vi "Host Access Control (SubVI).vi"(8 "Master /slave":bool, 10 "System Down?":bool, 11 "Data Cluster in":T1={"VI References"=[], "Addresses"=[], "Pilot"=FALSE, "DO Data"=[], "Access Restricted?"=FALSE, "Pilot Control References"=[], "CoPilot Control References"=[], "cRIO Config"=[], "datalog Q"=refnum, "PS_P"={"AI"=[], "DI"=[], "DO"=[], "Serial"=[], "CPU"={"Total Load"=[], "Interrupt Load"=[], "Total Physical"=0.0, "Free Physical"=0.0, "Primary Disk Capacity"=0.0, "Primary Disk Free"=0.0}, "Stop"=FALSE, "DO Channel"=[]}, "PS_S"={"AI"=[], "DI"=[], "DO"=[], "Serial"=[], "CPU"={"Total Load"=[], "Interrupt Load"=[], "Total Physical"=0.0, "Free Physical"=0.0, "Primary Disk Capacity"=0.0, "Primary Disk Free"=0.0}, "Stop"=FALSE, "DO Channel"=[]}, "IDE_P"={"AI"=[], "DI"=[], "DO"=[], "Serial"=[], "CPU"={"Total Load"=[], "Interrupt Load"=[], "Total Physical"=0.0, "Free Physical"=0.0, "Primary Disk Capacity"=0.0, "Primary Disk Free"=0.0}, "Stop"=FALSE, "DO Channel"=[]}, "IDE_S"={"AI"=[], "DI"=[], "DO"=[], "Serial"=[], "CPU"={"Total Load"=[], "Interrupt Load"=[], "Total Physical"=0.0, "Free Physical"=0.0, "Primary Disk Capacity"=0.0, "Primary Disk Free"=0.0}, "Stop"=FALSE, "DO Channel"=[]}, "PDE_P"={"AI"=[], "DI"=[], "DO"=[], "Serial"=[], "CPU"={"Total Load"=[], "Interrupt Load"=[], "Total Physical"=0.0, "Free Physical"=0.0, "Primary Disk Capacity"=0.0, "Primary Disk Free"=0.0}, "Stop"=FALSE, "DO Channel"=[]}, "PDE_S"={"AI"=[], "DI"=[], "DO"=[], "Serial"=[], "CPU"={"Total Load"=[], "Interrupt Load"=[], "Total Physical"=0.0, "Free Physical"=0.0, "Primary Disk Capacity"=0.0, "Primary Disk Free"=0.0}, "Stop"=FALSE, "DO Channel"=[]}, "GUI References"={"Control Names"=[], "Control References"=[]}, "GUI Data"=[], "TCP - Serial"=[], "TCP-Serial Q"=refnum, "TCP Serial Ref"=[], "Data Sets"=[], "Last Data"=[], "Alarm Data"=[], "DI Data"=[], "Ack Data"=[], "Buzzer Data"=[], "Pilot DO"=[], "Co-Pilot DO"=[], "System Down?"=FALSE, "Log Data"=[], "Update Array"=[], "MCC Data Log"=[], "MCC Data Not"=refnum, "Thruster control"=[refnum, refnum, refnum, refnum, refnum, refnum, refnum, refnum, refnum], "waga notifier out"=refnum, "Wago  log"=[], "Thruster Cont"=[0.0, 0.0, 0.0, 0.0, 0.0, 0.0, 0.0, 0.0, 0.0], "Cam Cont"=[FALSE, FALSE, FALSE, FALSE, FALSE, TRUE], "PDE_P TH Cont"={"COM 10"=0.0, "COM 11"=0.0, "COM 12"=0.0, "COM 13"=0.0}, "PDE_S TH Cont"={"COM 10"=0.0, "COM 11"=0.0, "COM 12"=0.0, "COM 13"=0.0}} {"cRIO Config"."AI"."Interface Data"."Timing"."sample mode" items=["Finite Samples"=10178, "Continuous Samples"=10123, "Hardware Timed Single Point"=12522]; "cRIO Config"."Async"."Interface Data"."Data"."Minor Frame Count" min=5 max=8 step=1}) -> ()   [LabVIEW 2021]
doc: "Control acess will be define here based on the Master or slave status & System Done Status which det from the Watch Dog UDP vi"
uses:
  Controls/Host - GUI Data Cluster.ctl
  Analog Output/Controls/AO JSON Data Cluster.ctl
  Analog Output/Controls/AO Interface Data Cluster.ctl
  Analog Output/Controls/AO Channel Configuration Cluster.ctl
  Analog Output/Controls/AO Timing Cluster.ctl
  Digital Output/Controls/DIO Configuration cluster.ctl
  Digital Output/Controls/DIO Interface Data.ctl
  Digital Output/SubVIs/Digital Dynamic Cluster.ctl
  Async JSON Cluster.ctl
  Async Interface Data Cluster.ctl
  Async Serial/Controls/Async Serial Configuration Cluster.ctl
  Async Serial/Controls/Async Frame Info Cluster.ctl
  Async Serial/Controls/Async Message Info Cluster.ctl
  Controls/Host Data Cluster.ctl
  Main Engine/Controls/Main Engine CPU Info.ctl
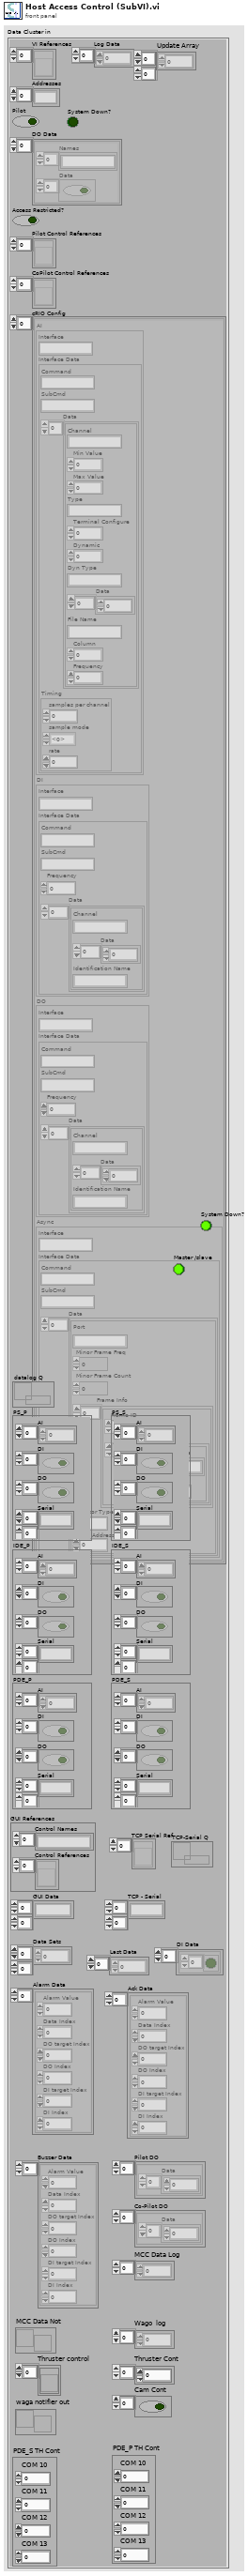
[diagram p1: front panel]
types:
  T1 = typedef "Host - GUI Data Cluster.ctl" = cluster{"VI References":refnum<vi>[], "Addresses":string[], "Pilot":bool, "DO Data":cluster{"Names":string[], "Data":bool[]}[], "Access Restricted?":bool, "Pilot Control References":refnum<vi>[], "CoPilot Control References":refnum<vi>[], "cRIO Config":cluster{"AI":T2, "DI":T6, "DO":T6, "Async":T9}[], "datalog Q":refnum<queue>, "PS_P":T14, "PS_S":T14, "IDE_P":T14, "IDE_S":T14, "PDE_P":T14, "PDE_S":T14, "GUI References":cluster{"Control Names":string[], "Control References":refnum<vi>[]}, "GUI Data":string[][], "TCP - Serial":string[][], "TCP-Serial Q":refnum<queue>, "TCP Serial Ref":refnum<vi>[], "Data Sets":dbl[][], "Last Data":dbl[], "Alarm Data":cluster{"Alarm Value":dbl, "Data Index":i32, "DO target Index":i32, "DO Index":i32, "DI target Index":i32, "DI Index":i32}[], "DI Data":cluster{bool[]}[], "Ack Data":cluster{"Alarm Value":dbl, "Data Index":i32, "DO target Index":i32, "DO Index":i32, "DI target Index":i32, "DI Index":i32}[], "Buzzer Data":cluster{"Alarm Value":dbl, "Data Index":i32, "DO target Index":i32, "DO Index":i32, "DI target Index":i32, "DI Index":i32}[], "Pilot DO":cluster{"Data":i32[]}[], "Co-Pilot DO":cluster{"Data":i32[]}[], "System Down?":bool, "Log Data":dbl[], "Update Array":i32[][], "MCC Data Log":dbl[], "MCC Data Not":refnum<notifier>, "Thruster control":refnum<vi>[], "waga notifier out":refnum<notifier>, "Wago  log":sgl[], "Thruster Cont":dbl[], "Cam Cont":bool[], "PDE_P TH Cont":cluster{"COM 10":dbl, "COM 11":dbl, "COM 12":dbl, "COM 13":dbl}, "PDE_S TH Cont":cluster{"COM 10":dbl, "COM 11":dbl, "COM 12":dbl, "COM 13":dbl}}
  T2 = typedef "AO JSON Data Cluster.ctl" = cluster{"Interface":string, "Interface Data":T3}
  T3 = typedef "AO Interface Data Cluster.ctl" = cluster{"Command":string, "SubCmd":string, "Data":T4[], "Timing":T5}
  T4 = typedef "AO Channel Configuration Cluster.ctl" = cluster{"Channel":string, "Min Value":dbl, "Max Value":dbl, "Type":string, "Terminal Configure":u16, "Dynamic":u8, "Dyn Type":string, "Data":dbl[], "File Name":string, "Column":i32, "Frequency":dbl}
  T5 = typedef "AO Timing Cluster.ctl" = cluster{"samples per channel":i32, "sample mode":i32, "rate":dbl}
  T6 = typedef "DIO Configuration cluster.ctl" = cluster{"Interface":string, "Interface Data":T7}
  T7 = typedef "DIO Interface Data.ctl" = cluster{"Command":string, "SubCmd":string, "Frequency":u16, "Data":T8[]}
  T8 = typedef "Digital Dynamic Cluster.ctl" = cluster{"Channel":string, "Data":u8[], "Identification Name":string}
  T9 = typedef "Async JSON Cluster.ctl" = cluster{"Interface":string, "Interface Data":T10}
  T10 = typedef "Async Interface Data Cluster.ctl" = cluster{"Command":string, "SubCmd":string, "Data":T11[]}
  T11 = typedef "Async Serial Configuration Cluster.ctl" = cluster{"Port":string, "Minor Frame Freq":u16, "Minor Frame Count":u16, "Frame Info":T12[], "Sensor Type":u16, "OIM Address":u16}
  T12 = typedef "Async Frame Info Cluster.ctl" = cluster{"Frame ID":u16, "Message Info":T13[]}
  T13 = typedef "Async Message Info Cluster.ctl" = cluster{"Message":u8[], "Message Name":string}
  T14 = typedef "Host Data Cluster.ctl" = cluster{"AI":dbl[], "DI":bool[], "DO":bool[], "Serial":string[][], "CPU":T15, "Stop":bool, "DO Channel":string[]}
  T15 = typedef "Main Engine CPU Info.ctl" = cluster{"Total Load":u32[], "Interrupt Load":u32[], "Total Physical":dbl, "Free Physical":dbl, "Primary Disk Capacity":dbl, "Primary Disk Free":dbl}
  T16 = enum8{"Enabled", "Disabled", "Disabled and Grayed Out"}
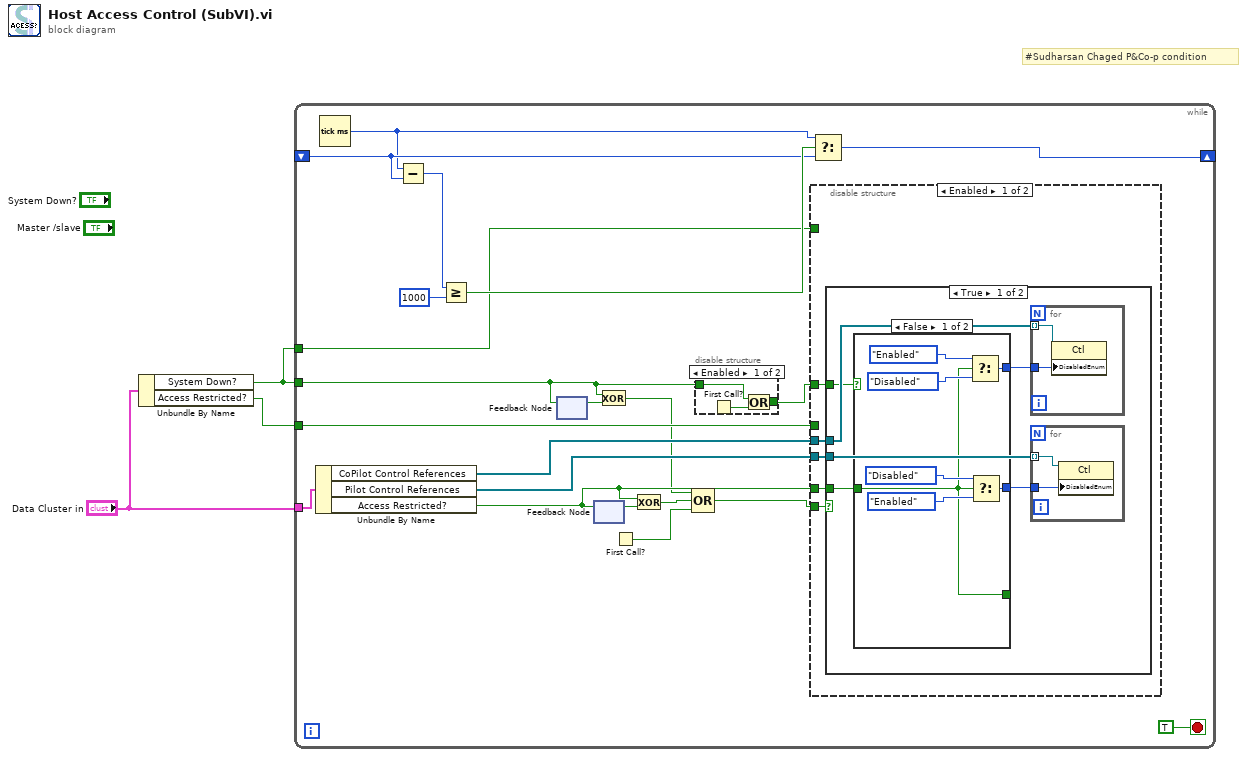
[diagram p0: block diagram]
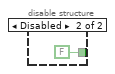
[diagram p2: hidden frame]
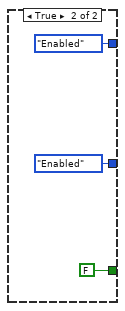
[diagram p3: hidden frame]
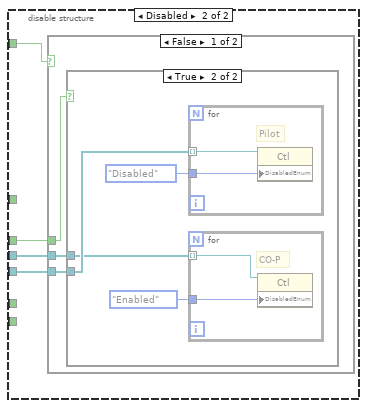
[diagram p5: hidden frame]
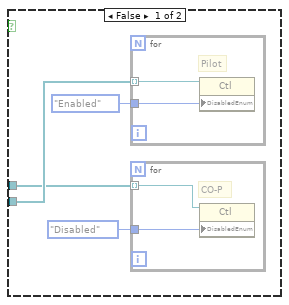
[diagram p6: hidden frame]
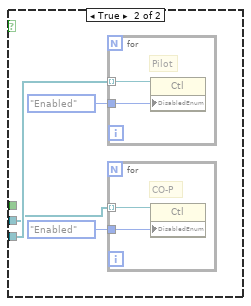
[diagram p7: hidden frame]
diagram:
  # "#Sudharsan Chaged P&Co-p condition"
  n1 = Unbundle By Name("Data Cluster in") -> ("System Down?"=w2:bool, "Access Restricted?"=w1:bool)
  n2 = while {
    tunnel: "Data Cluster in" -> [w24]
    shift-right: [w14] -> _
    shift-left: _ -> [w16]
    tunnel: w2 -> [w5]
    tunnel: w2 -> [w11]
    tunnel: w1 -> [w10]
    stop <- TRUE stop-if-true
    n3 = Unbundle By Name(w24) -> ("CoPilot Control References"=w22:refnum<vi>[], "Pilot Control References"=w23:refnum<vi>[], "Access Restricted?"=w9:bool)
    n4 = Tick Count (ms)() -> (millisecond timer value=w15:u32)
    n5 = Subtract(x=w15, y=w16) -> (x-y=w19:u32)
    n6 = Greater Or Equal?(x=w19, y=u32 1000) -> (x >= y?=w17:bool)
    n7 = feedback #1() -> (w12:bool)  [unwired: 1 in]
    n8 = feedback-in #1(w5) -> ()
    n9 = feedback-in #2(w9) -> ()
    n10 = feedback #2() -> (w13:bool)  [unwired: 1 in]
    n11 = Exclusive Or(1:w12, 2:w5) -> (0:w7:bool)
    n12 = First Call?() -> (First Call?: T/F=w21:bool)
    n13 = Exclusive Or(1:w13, 2:w9) -> (0:w8:bool)
    n14 = Compound Arithmetic op=OR(w7, w8, w21) -> (w6:bool)
    n15 = disable-structure shown="Enabled" {
      disable-tunnel: w5 -> [w26 _]
      disable-tunnel: [w25 FALSE] -> w4
      frame Enabled {
        n16 = First Call?() -> (First Call?: T/F=w27:bool)
        n17 = Or(x=w26, y=w27) -> (x .or. y?=w25:bool)
      }
      frame Disabled {
      }
    }
    n18 = disable-structure shown="Enabled" {
      disable-tunnel: w23 -> [w33 w55]
      disable-tunnel: w22 -> [w32 w54]
      disable-tunnel: w6 -> [w31 _]
      disable-tunnel: w9 -> [w30 _]
      disable-tunnel: w4 -> [w29 _]
      disable-tunnel: w11 -> [_ w57]
      disable-tunnel: w10 -> [_ w56]
      frame Enabled {
        n19 = case shown="True" w31 {
          tunnel: w33 -> [w39 _]
          tunnel: w30 -> [w35 _]
          tunnel: w32 -> [w36 _]
          tunnel: w29 -> [w34 _]
          frame True {
            n20 = case shown="False" w34 {
              tunnel: [w45 T16."Enabled" ("Disabled")] -> w38
              tunnel: [w43 T16."Enabled" ("t")] -> w37
              tunnel: w35 -> [w40 _]
              tunnel: [w40 FALSE ("Indicator")] -> _
              frame False {
                n21 = Select(t=T16."Enabled" ("Disabled"), s=w40, f=T16."Disabled" ("t")) -> (s? t:f=w43:T16)
                n22 = Select(t=T16."Disabled", s=w40, f=T16."Enabled" ("Disabled")) -> (s? t:f=w45:T16)
              }
              frame True {
              }
            }
            n23 = for {
              tunnel: w36 -> [w51] mode=indexing
              tunnel: w37 -> [w50]
              n24 = property class="Ctl"(reference=w51, "DisabledEnum"=w50) -> ()  [unwired: 1 in, 2 out]
            }
            n25 = for {
              tunnel: w39 -> [w53] mode=indexing
              tunnel: w38 -> [w52]
              n26 = property class="Ctl"(reference=w53, "DisabledEnum"=w52) -> ()  [unwired: 1 in, 2 out]
            }
          }
          frame False {
          }
        }
      }
      frame Disabled {
        n27 = case shown="False" w57 {
          tunnel: w56 -> [w60 _]
          tunnel: w55 -> [w59 w78]
          tunnel: w54 -> [w58 w77]
          frame False {
            n28 = case shown="True" w60 {
              tunnel: w59 -> [w62 w70]
              tunnel: w58 -> [w61 w69]
              frame False {
                n29 = for {
                  tunnel: T16."Enabled" ("Disabled") -> [w66]
                  tunnel: w62 -> [w65] mode=indexing
                  # "Pilot"
                  n30 = property class="Ctl"(reference=w65, "DisabledEnum"=w66) -> ()  [unwired: 1 in, 2 out]
                }
                n31 = for {
                  tunnel: T16."Disabled" ("t") -> [w68]
                  tunnel: w61 -> [w67] mode=indexing
                  # "CO-P"
                  n32 = property class="Ctl"(reference=w67, "DisabledEnum"=w68) -> ()  [unwired: 1 in, 2 out]
                }
              }
              frame True {
                n33 = for {
                  tunnel: T16."Disabled" ("Disabled") -> [w74]
                  tunnel: w70 -> [w73] mode=indexing
                  # "Pilot"
                  n34 = property class="Ctl"(reference=w73, "DisabledEnum"=w74) -> ()  [unwired: 1 in, 2 out]
                }
                n35 = for {
                  tunnel: T16."Enabled" ("t") -> [w76]
                  tunnel: w69 -> [w75] mode=indexing
                  # "CO-P"
                  n36 = property class="Ctl"(reference=w75, "DisabledEnum"=w76) -> ()  [unwired: 1 in, 2 out]
                }
              }
            }
          }
          frame True {
            n37 = for {
              tunnel: T16."Enabled" ("Disabled") -> [w82]
              tunnel: w78 -> [w81] mode=indexing
              # "Pilot"
              n38 = property class="Ctl"(reference=w81, "DisabledEnum"=w82) -> ()  [unwired: 1 in, 2 out]
            }
            n39 = for {
              tunnel: T16."Enabled" ("t") -> [w84]
              tunnel: w77 -> [w83] mode=indexing
              # "CO-P"
              n40 = property class="Ctl"(reference=w83, "DisabledEnum"=w84) -> ()  [unwired: 1 in, 2 out]
            }
          }
        }
      }
    }
    n41 = Select(t=w15, s=w17, f=w16) -> (s? t:f=w14:u32)
  }
